vi "Sub-VI_Erros-Som.vi"(10 "Nº de erros":dbl, 11 "Boolean in":bool) -> (3 "Nº de erros":dbl)   [LabVIEW 2019]
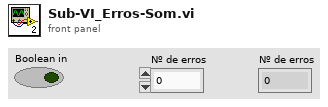
[diagram p1: front panel]
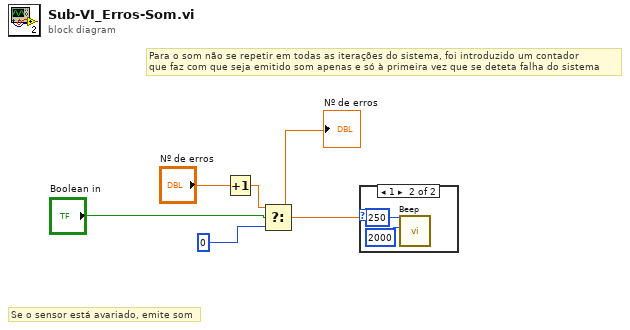
[diagram p0: block diagram]
diagram:
  # "Para o som não se repetir em todas as iterações do sistema, foi introduzido um contador\nque faz com que seja emitido som apenas e só à primeira vez que se deteta falha do sistema"
  # "Se o sensor está avariado, emite som"
  n1 = Increment(x="Nº de erros") -> (x+1=w5:dbl)
  n2 = Select(t=w5, s="Boolean in", f=0) -> (s? t:f=w1:dbl)
  "Nº de erros" <- w1
  n3 = case shown="1" w1 {
    frame 0, Default {
    }
    frame 1 {
      n4 = call <vilib>:"Beep.vi"("duration (msec)"=2000, "frequency (Hz)"=250) -> ()  [unwired: 10 in]
    }
  }
